vi "changeColor.vi"(1 "Array":string[](array[string]), 2 "last response 2":refnum<vi>) -> (0 "last response":string)   [LabVIEW 2009]
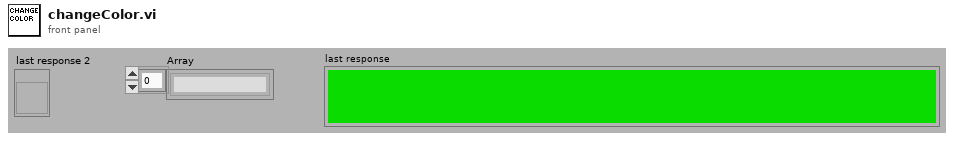
[diagram p1: front panel]
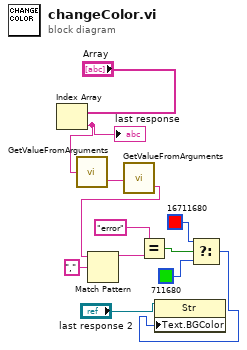
[diagram p0: block diagram]
diagram:
  n1 = Index Array(array="Array") -> (element=w2:string)  [unwired: 1 in]
  "last response" <- w2
  n2 = call "GetValueFromArguments.vi"("Arguments"=w2) -> ("Ip:port"=w3:string)  [unwired: 1 out]
  n3 = call "GetValueFromArguments.vi"("Arguments"=w3) -> ("Ip:port"=w4:string)  [unwired: 1 out]
  n4 = Match Pattern(string=w4, regular expression=",") -> (before substring=w6:string)  [unwired: 1 in, 3 out]
  n5 = Equal?(x="error", y=w6) -> (x = y?=w8:bool)
  n6 = Select(t=u32 16711680, s=w8, f=u32 711680) -> (s? t:f=w12:u32)
  n7 = property class="Str"(reference="last response 2", "Text.BGColor"=w12) -> ()  [unwired: 1 in, 2 out]
